vi "LVClass_CameraSet Get Default CameraParametersSetup.vi"(0 "CameraSet in":refnum<class "CameraSet.lvclass">, 11 "error in (no error)":errorcluster) -> (4 "CameraSet out":refnum<class "CameraSet.lvclass">, 6 "AllValueSetAndGet":T1[](array[typedef]), 8 "AllValueGet":T1[](array[typedef]), 10 "AllValueDisable":T1[](array[typedef]), 15 "error out":errorcluster)   [LabVIEW 2020, in "CameraSet.lvclass"]
uses:
  CameraSet.lvclass
  CameraParametersSetup.ctl
  CameraParameters_Type.ctl
  ParameterID.ctl
  CameraParameters_Authorization.ctl
  CameraParameters_OnFlyAuthorization.ctl
  CameraSet.lvclass/CameraSet.ctl
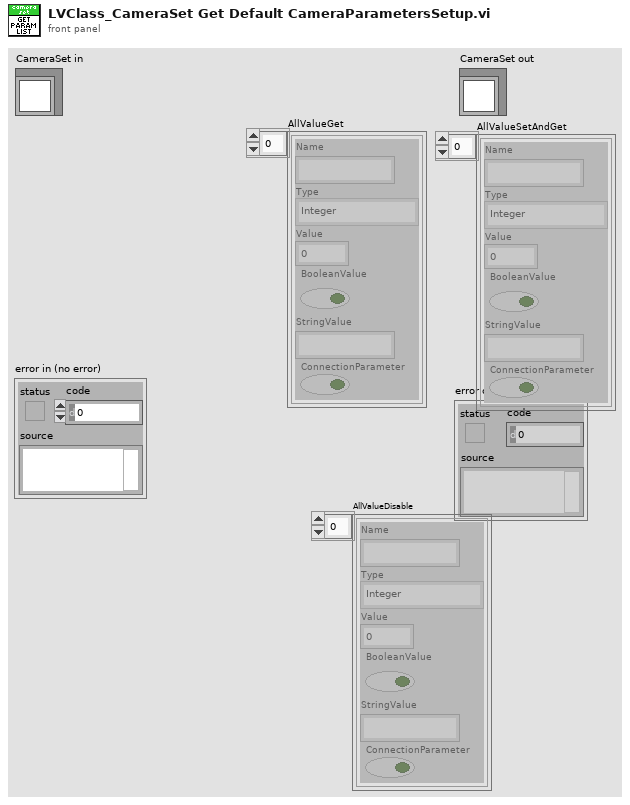
[diagram p1: front panel]
types:
  T1 = typedef "CameraParametersSetup.ctl" = cluster{"Name":string, "Type":T2, "Value":dbl, "BooleanValue":bool, "StringValue":string, "ConnectionParameter":bool}
  T2 = typedef "CameraParameters_Type.ctl" = enum16{"Integer", "Real", "String", "Boolean"}
  T3 = typedef "CameraParameters_Authorization.ctl" = enum16{"Disable", "Gettable", "Settable - Gettable"}
  T4 = typedef "CameraParameters_OnFlyAuthorization.ctl" = enum16{"None", "Gettable", "Settable", "Settable - Gettable"}
  T5 = typedef "ParameterID.ctl" = cluster{"Name":string, "ConnectionParameter?":bool, "Type":T2, "Authorization":T3, "OnFlyAuthorization":T4, "StringValue":string, "Value":dbl, "Min":dbl, "Max":dbl, "BooleanValue":bool, "StringParameterList":string[]}
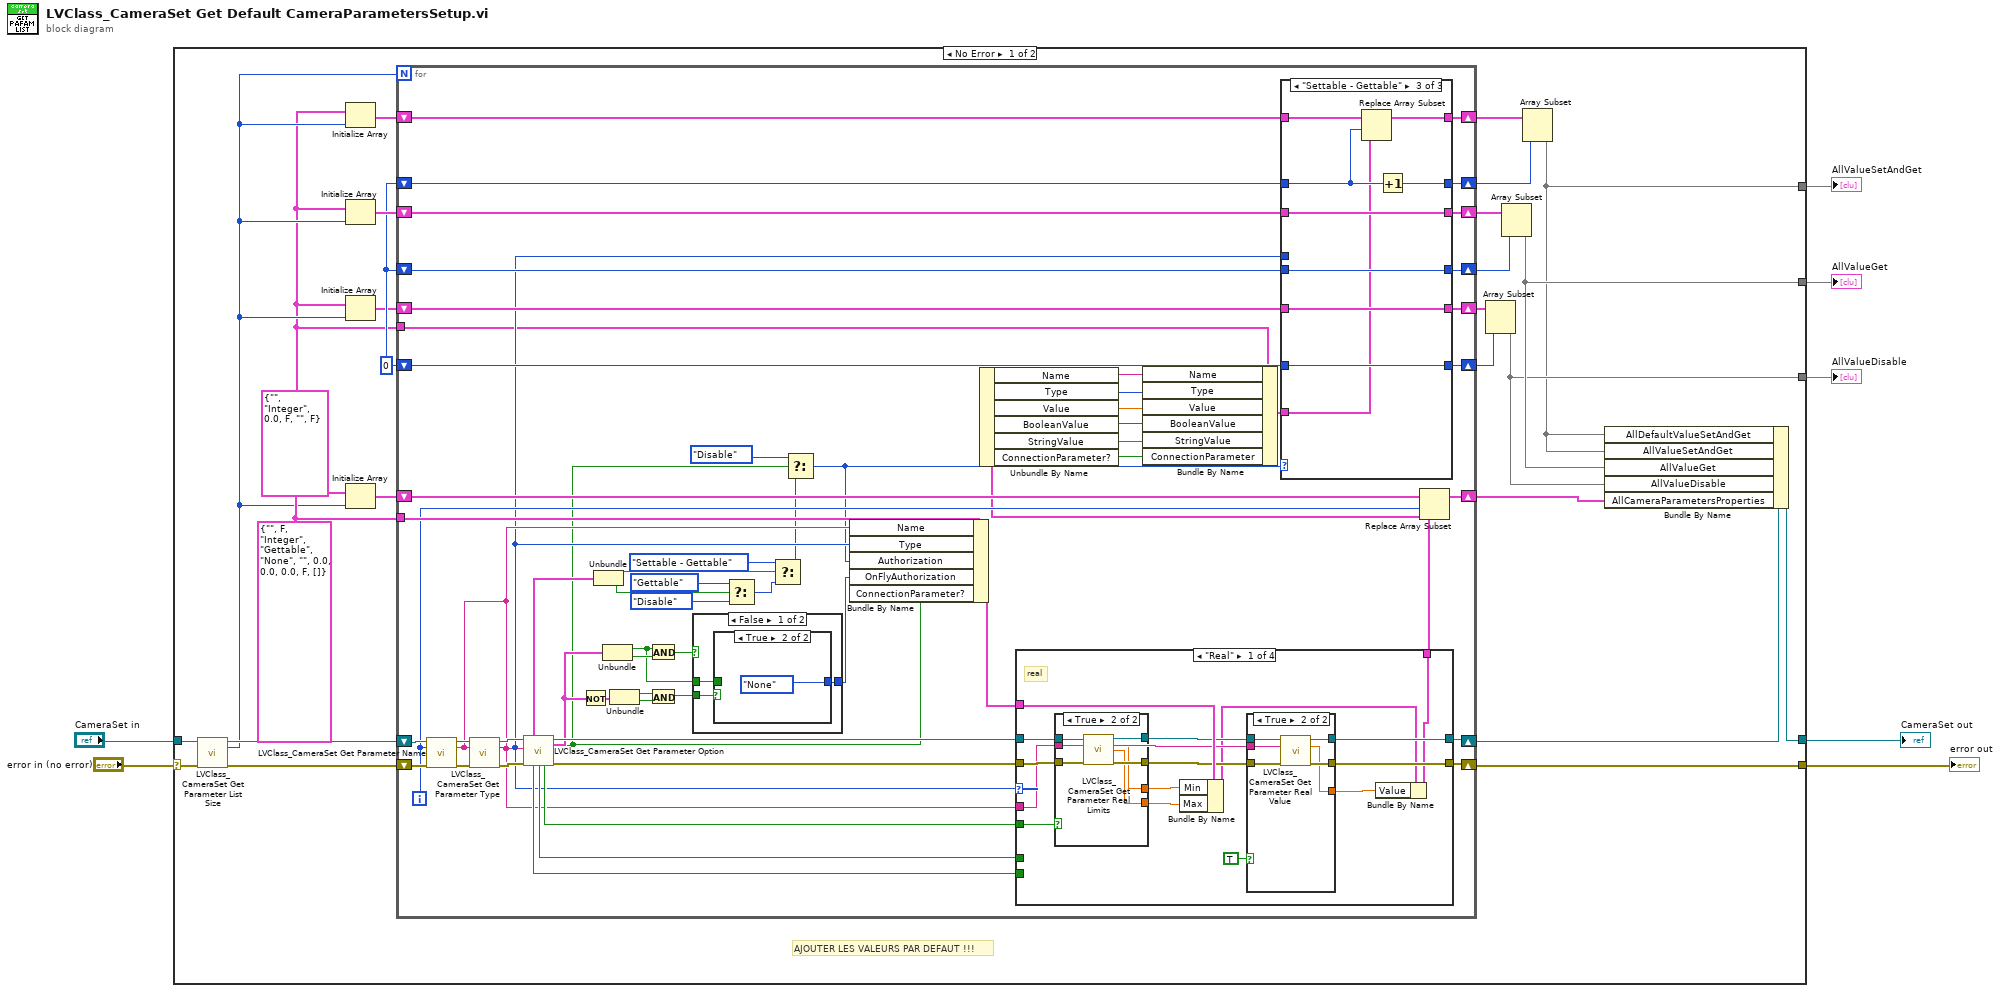
[diagram p0: block diagram]
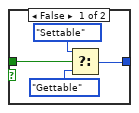
[diagram p2: hidden frame]
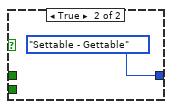
[diagram p3: hidden frame]
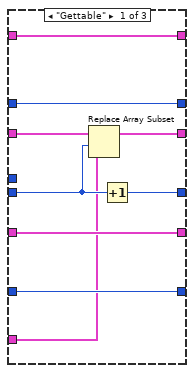
[diagram p4: hidden frame]
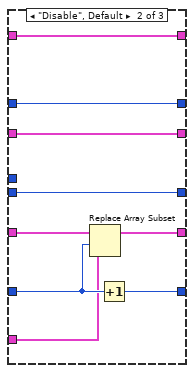
[diagram p5: hidden frame]
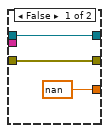
[diagram p6: hidden frame]
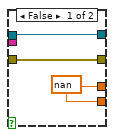
[diagram p7: hidden frame]
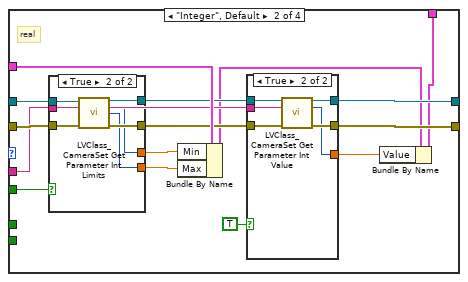
[diagram p8: hidden frame]
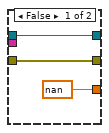
[diagram p9: hidden frame]
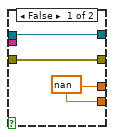
[diagram p10: hidden frame]
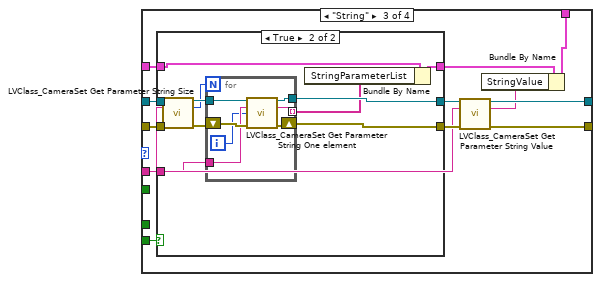
[diagram p11: hidden frame]
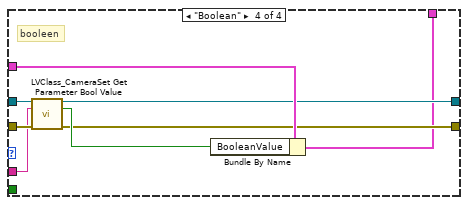
[diagram p13: hidden frame]
diagram:
  n1 = case shown="No Error" "error in (no error)" {
    selector: "error in (no error)" -> [w30 w240]
    tunnel: [w29 w240] -> w1
    tunnel: [w31 w239] -> w2
    tunnel: "CameraSet in" -> [w28 w239]
    tunnel: [w10 _] -> w5
    tunnel: [w8 _] -> w4
    tunnel: [w9 _] -> w3
    frame No Error {
      w13 = T1 {"Name"="", "Type"=enum."Integer", "Value"=0.0, "BooleanValue"=FALSE, "StringValue"="", "ConnectionParameter"=FALSE} ("CameraParametersSetup")
      w16 = 0
      w24 = T5 {"Name"="", "ConnectionParameter?"=FALSE, "Type"=enum."Integer", "Authorization"=enum."Gettable", "OnFlyAuthorization"=enum."None", "StringValue"="", "Value"=0.0, "Min"=0.0, "Max"=0.0, "BooleanValue"=FALSE, "StringParameterList"=[]} ("CameraParameters")
      # "AJOUTER LES VALEURS PAR DEFAUT !!!"
      n2 = call "LVClass_CameraSet Get Parameter List Size.vi"("CameraSet.lvclass"=w28, "error in (no error)"=w30) -> ("CameraSet.lvclass"=w27:refnum<class "CameraSet.lvclass">, "size"=w14:i32, "error out"=w32:errorcluster)  [unwired: 11 in]
      n3 = Initialize Array(w13, w14) -> (w19:T1[])
      n4 = Initialize Array(w13, w14) -> (w21:T1[])
      n5 = Initialize Array(w13, w14) -> (w15:T1[])
      n6 = Initialize Array(w24, w14) -> (w25:T5[])
      n7 = for {
        N: w14 -> [_]
        tunnel: w24 -> [w89]
        shift-right: [w88] -> w29
        shift-left: w32 -> [w92]
        shift-right: [w87] -> w26
        shift-left: w27 -> [w93]
        shift-right: [w75] -> w23
        shift-left: w25 -> [w76]
        shift-right: [w72] -> w20
        shift-left: w16 -> [w73]
        shift-right: [w71] -> w22
        shift-left: w21 -> [w70]
        shift-right: [w68] -> w18
        shift-left: w19 -> [w69]
        shift-right: [w66] -> w17
        shift-left: w16 -> [w67]
        shift-right: [w51] -> w11
        shift-left: w16 -> [w50]
        shift-right: [w48] -> w12
        shift-left: w15 -> [w49]
        tunnel: w13 -> [w38]
        i -> [w74]
        n8 = call "LVClass_CameraSet Get Parameter Name.vi"("CameraSet.lvclass"=w93, "index"=w74, "error in (no error)"=w92) -> ("CameraSet.lvclass"=w91:refnum<class "CameraSet.lvclass">, "parameter_name"=w47:string, "error out"=w90:errorcluster)  [unwired: 10 in]
        n9 = call "LVClass_CameraSet Get Parameter Type.vi"("CameraSet.lvclass"=w91, "parameter_name"=w47, "error in (no error)"=w90) -> ("CameraSet.lvclass"=w86:refnum<class "CameraSet.lvclass">, "Type"=w46:T2, "error out"=w85:errorcluster)  [unwired: 10 in]
        n10 = call "LVClass_CameraSet Get Parameter Option.vi"("CameraSet.lvclass"=w86, "parameter_name"=w47, "error in (no error)"=w85) -> ("Settable-Gettable?"=w63:cluster{"Settable":bool, "Gettable":bool}, "Settable-Gettable on fly?"=w56:cluster{"Settable":bool, "Gettable":bool}, "CameraSet.lvclass"=w84:refnum<class "CameraSet.lvclass">, "is_connection_parameter?"=w36:bool, "String enum"=w64:bool, "DefaultValueExist"=w65:bool, "minmax"=w77:bool, "error out"=w83:errorcluster)  [unwired: 5 in]
        n11 = Not(x=w56) -> (.not. x?=w54:cluster{"Settable":bool, "Gettable":bool})
        n12 = Unbundle(w63) -> ("Settable"=w62:bool, "Gettable"=w61:bool)
        n13 = Unbundle(w56) -> ("Settable"=w53:bool, "Gettable"=w60:bool)
        n14 = Unbundle(w54) -> ("Settable"=w55:bool, "Gettable"=w58:bool)
        n15 = And(x=w53, y=w60) -> (x .and. y?=w59:bool)
        n16 = And(x=w55, y=w58) -> (x .and. y?=w57:bool)
        n17 = case shown="False" w59 {
          tunnel: [w95 CameraParameters_OnFlyAuthorization."Settable - Gettable" ("OnFlyAuthorization")] -> w52
          tunnel: w57 -> [w96 _]
          tunnel: w53 -> [w94 _]
          frame False {
            n18 = case shown="True" w96 {
              tunnel: [w100 CameraParameters_OnFlyAuthorization."None" ("OnFlyAuthorization")] -> w95
              tunnel: w94 -> [w97 _]
              frame False {
                n19 = Select(t=CameraParameters_OnFlyAuthorization."Settable" ("OnFlyAuthorization"), s=w97, f=CameraParameters_OnFlyAuthorization."Gettable" ("OnFlyAuthorization")) -> (s? t:f=w100:T4)
              }
              frame True {
              }
            }
          }
          frame True {
          }
        }
        n20 = Select(t=CameraParameters_Authorization."Gettable" ("Authorization"), s=w61, f=CameraParameters_Authorization."Disable") -> (s? t:f=w80:T3)
        n21 = Select(t=CameraParameters_Authorization."Settable - Gettable", s=w62, f=w80) -> (s? t:f=w34:T3)
        n22 = Select(t=CameraParameters_Authorization."Disable" ("f"), s=w36, f=w34) -> (s? t:f=w33:T3)
        n23 = Bundle By Name(cluster=w89, "Name"=w47, "Type"=w46, "Authorization"=w33, "OnFlyAuthorization"=w52, "ConnectionParameter?"=w36) -> (w78:T5)
        n24 = case shown="\"Real\"" w46 {
          tunnel: w78 -> [w144 w178 w201 w237]
          tunnel: w47 -> [w138 w172 w203 w234]
          tunnel: [w135 w169 w205 w232] -> w88
          tunnel: w84 -> [w143 w177 w209 w236]
          tunnel: w83 -> [w142 w176 w208 w235]
          tunnel: [w134 w168 w206 w233] -> w87
          tunnel: w65 -> [_ _ _ _]
          tunnel: w77 -> [w141 w175 _ _]
          tunnel: w64 -> [_ _ w199 _]
          tunnel: [w132 w166 w198 w231] -> w45
          frame "Real" {
            # "real"
            n25 = case shown="True" w141 {
              tunnel: w138 -> [_ w163]
              tunnel: [w156 w162] -> w136
              tunnel: [w155 w161] -> w137
              tunnel: w143 -> [w155 w160]
              tunnel: w142 -> [w156 w159]
              tunnel: [w154 w158] -> w140
              tunnel: [w154 w157] -> w139
              frame False {
                w154 = nan ("f")
              }
              frame True {
                n26 = call "LVClass_CameraSet Get Parameter Real Limits.vi"("CameraSet.lvclass"=w160, "parameter_name"=w163, "error in (no error)"=w159) -> ("CameraSet.lvclass"=w161:refnum<class "CameraSet.lvclass">, "min"=w158:dbl, "max"=w157:dbl, "error out"=w162:errorcluster)  [unwired: 9 in]
              }
            }
            n27 = Bundle By Name(cluster=w144, "Min"=w140, "Max"=w139) -> (w133:T5)
            n28 = case shown="True" TRUE {
              tunnel: w138 -> [_ w153]
              tunnel: w137 -> [w147 w152]
              tunnel: w136 -> [w146 w151]
              tunnel: [w146 w150] -> w135
              tunnel: [w147 w149] -> w134
              tunnel: [nan ("f") w148] -> w131
              frame False {
              }
              frame True {
                n29 = call "LVClass_CameraSet Get Parameter Real Value.vi"("CameraSet.lvclass"=w152, "parameter_name"=w153, "error in (no error)"=w151) -> ("CameraSet.lvclass"=w149:refnum<class "CameraSet.lvclass">, "Value"=w148:dbl, "error out"=w150:errorcluster)  [unwired: 10 in]
              }
            }
            n30 = Bundle By Name(cluster=w133, "Value"=w131) -> (w132:T5)
          }
          frame "Integer", Default {
            # "real"
            n31 = case shown="True" w175 {
              tunnel: w172 -> [_ w197]
              tunnel: [w190 w196] -> w170
              tunnel: [w189 w195] -> w171
              tunnel: w177 -> [w189 w194]
              tunnel: w176 -> [w190 w193]
              tunnel: [w188 w192] -> w174
              tunnel: [w188 w191] -> w173
              frame False {
                w188 = nan ("f")
              }
              frame True {
                n32 = call "LVClass_CameraSet Get Parameter Int Limits.vi"("CameraSet.lvclass"=w194, "parameter_name"=w197, "error in (no error)"=w193) -> ("CameraSet.lvclass"=w195:refnum<class "CameraSet.lvclass">, "min"=w192:i32, "max"=w191:i32, "error out"=w196:errorcluster)  [unwired: 9 in]
              }
            }
            n33 = Bundle By Name(cluster=w178, "Min"=w174, "Max"=w173) -> (w167:T5)
            n34 = case shown="True" TRUE {
              tunnel: w172 -> [_ w187]
              tunnel: w171 -> [w181 w186]
              tunnel: w170 -> [w180 w185]
              tunnel: [w180 w184] -> w169
              tunnel: [w181 w183] -> w168
              tunnel: [nan ("f") w182] -> w165
              frame False {
              }
              frame True {
                n35 = call "LVClass_CameraSet Get Parameter Int Value.vi"("CameraSet.lvclass"=w186, "parameter_name"=w187, "error in (no error)"=w185) -> ("CameraSet.lvclass"=w183:refnum<class "CameraSet.lvclass">, "Value"=w182:i32, "error out"=w184:errorcluster)  [unwired: 10 in]
              }
            }
            n36 = Bundle By Name(cluster=w167, "Value"=w165) -> (w166:T5)
          }
          frame "String" {
            n37 = case shown="True" w199 {
              tunnel: w209 -> [w212 w223]
              tunnel: w208 -> [w211 w222]
              tunnel: [w212 w218] -> w207
              tunnel: [w211 w217] -> w204
              tunnel: w203 -> [_ w216]
              tunnel: w201 -> [w210 w215]
              tunnel: [w210 w213] -> w200
              frame False {
              }
              frame True {
                n38 = call "LVClass_CameraSet Get Parameter String Size.vi"("CameraSet.lvclass"=w223, "parameter name"=w216, "error in (no error)"=w222) -> ("CameraSet.lvclass"=w221:refnum<class "CameraSet.lvclass">, "size"=w219:i32, "error out"=w220:errorcluster)  [unwired: 10 in]
                n39 = for {
                  N: w219 -> [_]
                  tunnel: w216 -> [w228]
                  tunnel: [w225] -> w218
                  tunnel: w221 -> [w230]
                  shift-right: [w224] -> w217
                  shift-left: w220 -> [w229]
                  tunnel: [w226] -> w214 mode=indexing
                  i -> [w227]
                  n40 = call "LVClass_CameraSet Get Parameter String One element.vi"("CameraSet.lvclass"=w230, "parameter name"=w228, "index"=w227, "error in (no error)"=w229) -> ("CameraSet.lvclass"=w225:refnum<class "CameraSet.lvclass">, "value"=w226:string, "error out"=w224:errorcluster)  [unwired: 9 in]
                }
                n41 = Bundle By Name(cluster=w215, "StringParameterList"=w214) -> (w213:T5)
              }
            }
            n42 = call "LVClass_CameraSet Get Parameter String Value.vi"("CameraSet.lvclass"=w207, "parameter name"=w203, "error in (no error)"=w204) -> ("CameraSet.lvclass"=w206:refnum<class "CameraSet.lvclass">, "Default value"=w202:string, "error out"=w205:errorcluster)  [unwired: 10 in]
            n43 = Bundle By Name(cluster=w200, "StringValue"=w202) -> (w198:T5)
          }
          frame "Boolean" {
            # "booleen"
            n44 = call "LVClass_CameraSet Get Parameter Bool Value.vi"("CameraSet.lvclass"=w236, "parameter_name"=w234, "error in (no error)"=w235) -> ("CameraSet.lvclass"=w233:refnum<class "CameraSet.lvclass">, "Value"=w238:bool, "error out"=w232:errorcluster)  [unwired: 10 in]
            n45 = Bundle By Name(cluster=w237, "BooleanValue"=w238) -> (w231:T5)
          }
        }
        n46 = Unbundle By Name(w45) -> ("Name"=w44:string, "Type"=w43:T2, "Value"=w42:dbl, "BooleanValue"=w41:bool, "StringValue"=w40:string, "ConnectionParameter?"=w37:bool)
        n47 = Bundle By Name(cluster=w38, "Name"=w44, "Type"=w43, "Value"=w42, "BooleanValue"=w41, "StringValue"=w40, "ConnectionParameter"=w37) -> (w39:T1)
        n48 = case shown="\"Settable - Gettable\"" w33 {
          tunnel: w73 -> [w111 w114 w124]
          tunnel: [w110 w114 w124] -> w72
          tunnel: [w109 w113 w125] -> w71
          tunnel: w46 -> [_ _ _]
          tunnel: w70 -> [w108 w113 w125]
          tunnel: w69 -> [w106 w119 w129]
          tunnel: [w106 w119 w128] -> w68
          tunnel: w67 -> [w107 w120 w127]
          tunnel: [w107 w120 w126] -> w66
          tunnel: [w105 w118 w123] -> w51
          tunnel: w50 -> [w105 w117 w123]
          tunnel: w49 -> [w104 w116 w122]
          tunnel: [w104 w115 w122] -> w48
          tunnel: w39 -> [w103 w112 w121]
          frame "Gettable" {
            n49 = Replace Array Subset(array=w108, new element=w103, index=w111) -> (w109:T1[])
            n50 = Increment(x=w111) -> (x+1=w110:i32)
          }
          frame "Disable", Default {
            n51 = Replace Array Subset(array=w116, new element=w112, index=w117) -> (w115:T1[])
            n52 = Increment(x=w117) -> (x+1=w118:i32)
          }
          frame "Settable - Gettable" {
            n53 = Replace Array Subset(array=w129, new element=w121, index=w127) -> (w128:T1[])
            n54 = Increment(x=w127) -> (x+1=w126:i32)
          }
        }
        n55 = Replace Array Subset(array=w76, new element=w45, index=w74) -> (w75:T5[])
      }
      n56 = Array Subset(array=w12, length=w11) -> (w9:T1[])  [unwired: 1 in]
      n57 = Array Subset(array=w22, length=w20) -> (w10:T1[])  [unwired: 1 in]
      n58 = Array Subset(array=w18, length=w17) -> (w8:T1[])  [unwired: 1 in]
      n59 = Bundle By Name(cluster=w26, "AllDefaultValueSetAndGet"=w8, "AllValueSetAndGet"=w8, "AllValueGet"=w10, "AllValueDisable"=w9, "AllCameraParametersProperties"=w23) -> (w31:refnum<class "CameraSet.lvclass">)
    }
    frame Error {
    }
  }
  "error out" <- w1
  "CameraSet out" <- w2
  "AllValueGet" <- w5
  "AllValueSetAndGet" <- w4
  "AllValueDisable" <- w3
